vi "hamamatsuBuffer.vi"(0 "action":u16(ring) items=["init", "read", "read stack", "write"], 1 "frameIn":u16[][](array[numeric]), 2 "index":i32, 3 "indexes":i32[](array[numeric]), 4 "frameBufferIn":u16[][][](array[numeric])) -> (5 "frameOut":u16[][](array[numeric]), 6 "stackOut":u16[][][](array[numeric]))   [LabVIEW 2017]
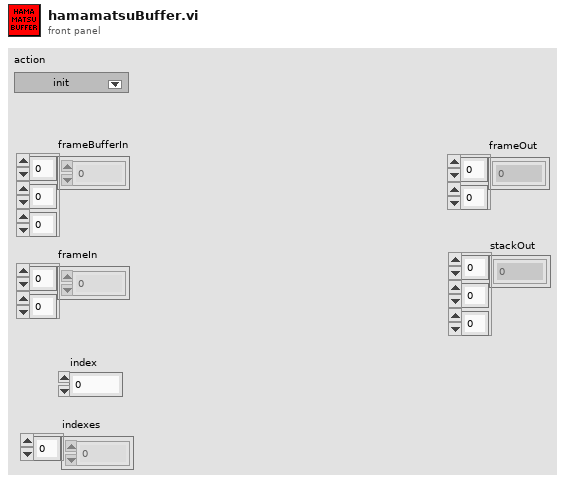
[diagram p1: front panel]
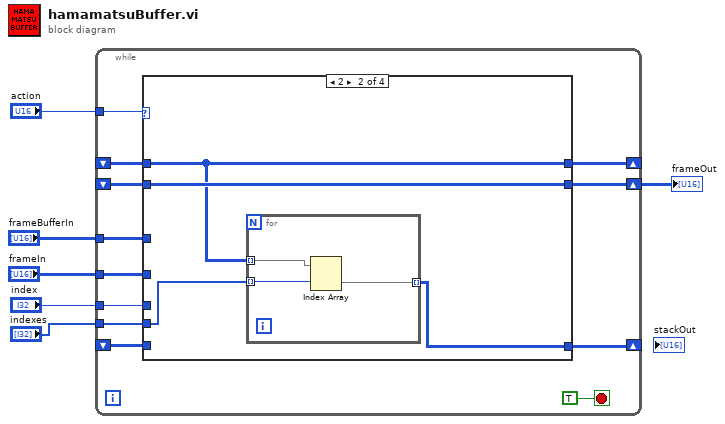
[diagram p0: block diagram]
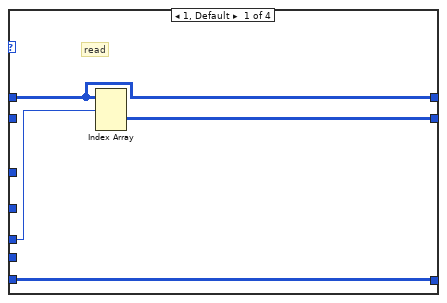
[diagram p2: hidden frame]
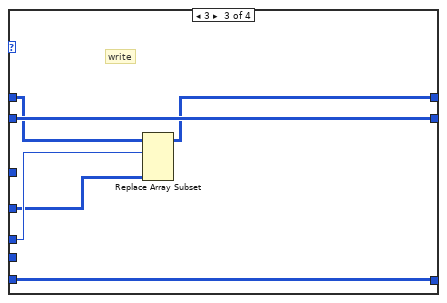
[diagram p3: hidden frame]
diagram:
  n1 = while {
    shift-right: [w15] -> _
    shift-left: _ -> [w12]
    tunnel: "frameBufferIn" -> [w16]
    tunnel: "action" -> [w17]
    tunnel: "index" -> [w14]
    tunnel: "frameIn" -> [w13]
    shift-right: [w11] -> w2
    shift-left: _ -> [w10]
    shift-right: [w9] -> _
    shift-left: _ -> [w8]
    tunnel: "indexes" -> [w7]
    stop <- TRUE stop-if-true
    n2 = case shown="2" w17 {
      tunnel: w16 -> [_ _ _ w38]
      tunnel: [w20 w24 w31 w38] -> w15
      tunnel: w14 -> [w22 _ w33 _]
      tunnel: w13 -> [_ _ w32 _]
      tunnel: w12 -> [w20 w24 w34 _]
      tunnel: [w21 w26 w35 w37] -> w11
      tunnel: w10 -> [_ w26 w35 w37]
      tunnel: [w19 w23 w30 w36] -> w9
      tunnel: w8 -> [w19 _ w30 w36]
      tunnel: w7 -> [_ w25 _ _]
      frame 1, Default {
        # "read"
        n3 = Index Array(array=w20, index (dim 0)=w22) -> (element=w21:u16[][])  [unwired: 2 in]
      }
      frame 2 {
        n4 = for {
          tunnel: w25 -> [w28] mode=indexing
          tunnel: w24 -> [w29] mode=indexing
          tunnel: [w27] -> w23 mode=indexing
          n5 = Index Array(array=w29, index (row)=w28) -> (element=w27:u16[])  [unwired: 1 in]
        }
      }
      frame 3 {
        # "write"
        n6 = Replace Array Subset(array=w34, new element=w32, index (dim 0)=w33) -> (w31:u16[][][])  [unwired: 2 in]
      }
      frame 0 {
        # "init"
      }
    }
  }
  "frameOut" <- w2
